vi "Nota_Frecventa.vi"(10 "Nota Muzicala":T1(ring)) -> (2 "Frecventa (Hz)":dbl)   [LabVIEW 2026]
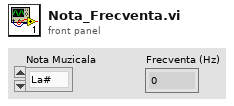
[diagram p1: front panel]
types:
  T1 = enum16{"La#", "Sol#", "Fa#", "Re#", "Do#", "Do_sus", "Si", "La", "Sol", "Fa", "Mi", "Re", "Do"}
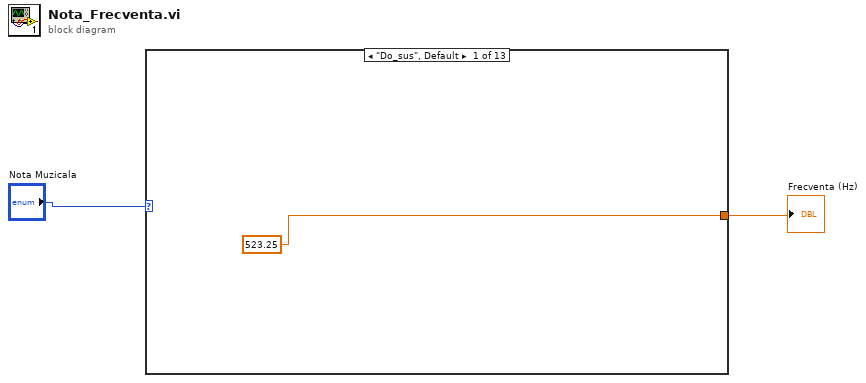
[diagram p0: block diagram]
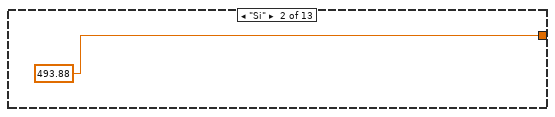
[diagram p2: hidden frame]
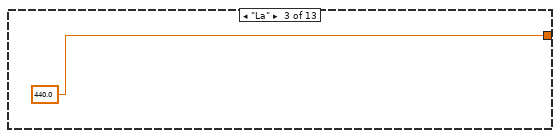
[diagram p3: hidden frame]
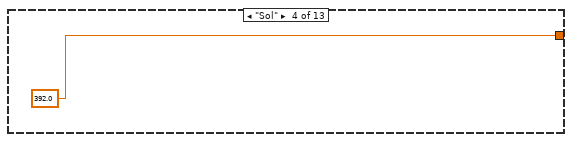
[diagram p4: hidden frame]
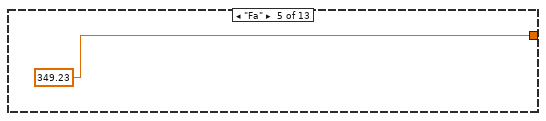
[diagram p5: hidden frame]
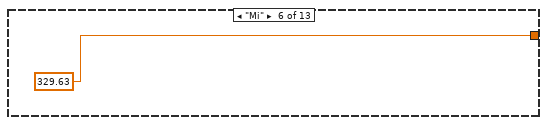
[diagram p6: hidden frame]
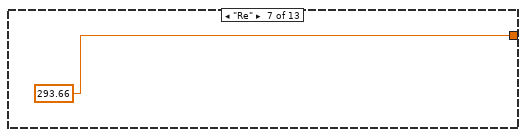
[diagram p7: hidden frame]
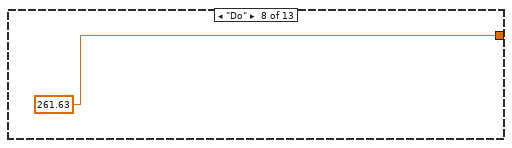
[diagram p8: hidden frame]
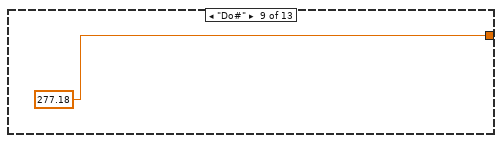
[diagram p9: hidden frame]
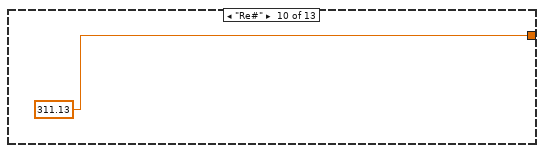
[diagram p10: hidden frame]
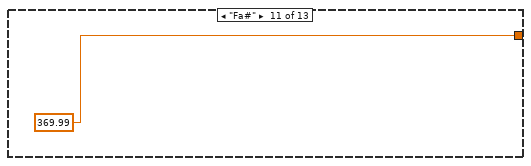
[diagram p11: hidden frame]
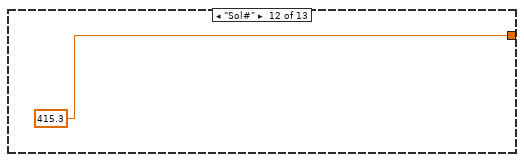
[diagram p12: hidden frame]
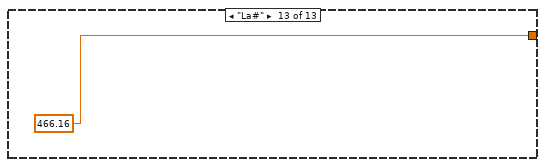
[diagram p13: hidden frame]
diagram:
  n1 = case shown="\"Do_sus\", Default" "Nota Muzicala" {
    tunnel: [523.25 493.88 440.0 392.0 349.23 329.63 293.66 261.63 277.18 311.13 369.99 415.3 466.16] -> w2
    frame "Do_sus", Default {
    }
    frame "Si" {
    }
    frame "La" {
    }
    frame "Sol" {
    }
    frame "Fa" {
    }
    frame "Mi" {
    }
    frame "Re" {
    }
    frame "Do" {
    }
    frame "Do#" {
    }
    frame "Re#" {
    }
    frame "Fa#" {
    }
    frame "Sol#" {
    }
    frame "La#" {
    }
  }
  "Frecventa (Hz)" <- w2
